vi "Get Wheel Information_Caster.vi"(8 "error in (no error)":errorcluster, 11 "caster wheel in":refnum<class "NI_Robotics_Caster Wheel.lvclass">) -> (0 "error out":errorcluster, 1 "wheel name":string, 2 "wheel parameters":T1={"wheel radius"=1.0, "gear ratio"=1.0, "forward rotation direction"=0} {"forward rotation direction" items=["Clockwise", "Counterclockwise"]}, 3 "caster wheel out":refnum<class "NI_Robotics_Caster Wheel.lvclass">, 4 "motor communication":refnum<class "NI_Robotics_Motor Communication.lvclass">, 5 "caster parameters":T3={"forward offset"=0.0, "caster gear ratio"=1.0}, 6 "caster motor communication":refnum<class "NI_Robotics_Motor Communication.lvclass">)   [LabVIEW 2017, in "NI_Robotics_Caster Wheel.lvclass"]
doc: "Returns information, such as <B>wheel radius</B> and <B>gear ratio</B>, for the wheel you specify. You must manually select the polymorphic instance to use."
uses:
  <vilib>/robotics/Steering/Caster Wheel/NI_Robotics_Caster Wheel.lvclass
  c:/Program Files (x86)/National Instruments/LabVIEW 2017/vi.lib/robotics/Steering/Wheel/NI_Robotics_Wheel.lvclass
  <vilib>/robotics/Steering/Caster Wheel/Caster Wheel Parameters.ctl
  <vilib>/robotics/Steering/Wheel/Wheel Parameters.ctl
  <vilib>/robotics/Steering/Wheel/Rotation Direction.ctl
  <vilib>/robotics/Actuation/Motor Communication/NI_Robotics_Motor Communication.lvclass
  <vilib>/robotics/Steering/Caster Wheel/NI_Robotics_Caster Wheel.lvclass/NI_Robotics_Caster Wheel.ctl
  <vilib>/robotics/Steering/Wheel/NI_Robotics_Wheel.lvclass/NI_Robotics_Wheel.ctl
  <vilib>/robotics/Steering/Wheel/NI_Robotics_Wheel.lvclass
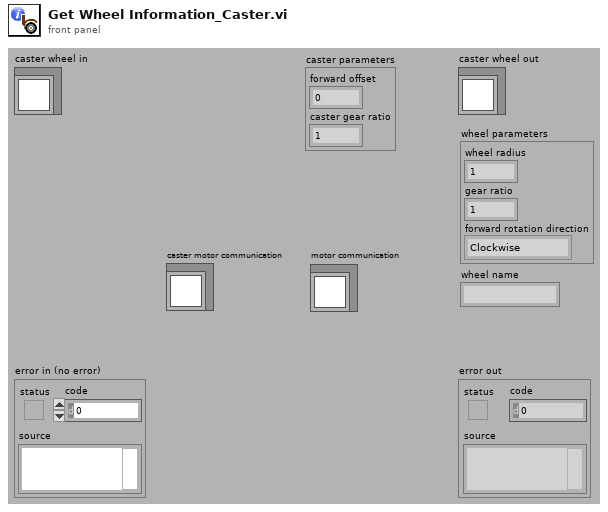
[diagram p1: front panel]
types:
  T1 = typedef "NI_Robotics_Wheel.lvclass/Wheel Parameters.ctl" = cluster{"wheel radius":dbl, "gear ratio":dbl, "forward rotation direction":T2}
  T2 = typedef "NI_Robotics_Wheel.lvclass/Rotation Direction.ctl" = u16
  T3 = typedef "NI_Robotics_Caster Wheel.lvclass/Caster Wheel Parameters.ctl" = cluster{"forward offset":dbl, "caster gear ratio":dbl}
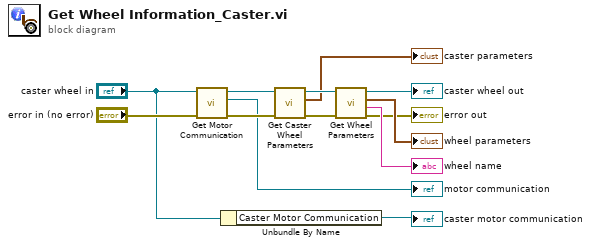
[diagram p0: block diagram]
diagram:
  n1 = call <vilib>:"Get Motor Communication.vi"("error in (no error)"="error in (no error)", "wheel in"="caster wheel in") -> ("error out"=w5:errorcluster, "motor communication"=→"motor communication":refnum<class "NI_Robotics_Motor Communication.lvclass">, "wheel out"=w13:refnum<class "NI_Robotics_Caster Wheel.lvclass">)  [unwired: 7 in]
  n2 = Unbundle By Name("caster wheel in") -> ("Caster Motor Communication"=→"caster motor communication":refnum<class "NI_Robotics_Motor Communication.lvclass">)
  n3 = call <vilib>:"Get Caster Wheel Parameters.vi"("error in (no error)"=w5, "caster wheel in"=w13) -> ("error out"=w7:errorcluster, "caster parameters"=→"caster parameters":T3, "caster wheel out"=w12:refnum<class "NI_Robotics_Caster Wheel.lvclass">)  [unwired: 7 in]
  n4 = call <vilib>:"Get Wheel Parameters.vi"("error in (no error)"=w7, "wheel in"=w12) -> ("error out"=→"error out":errorcluster, "wheel name"=→"wheel name":string, "wheel parameters"=→"wheel parameters":T1, "wheel out"=→"caster wheel out":refnum<class "NI_Robotics_Caster Wheel.lvclass">)  [unwired: 6 in]
